vi "manejadorErrores.vi"(8 "error in (no error)":errorcluster, 10 "Enc_values":T1) -> (0 "error out":errorcluster, 2 "Enc_values 2":T1)   [LabVIEW 2026]
uses:
  Control/Ctr_Enc_Values.ctl
  Control/Ctrl_Errores.ctl
  Control/Ctrl_Motores_Valores.ctl
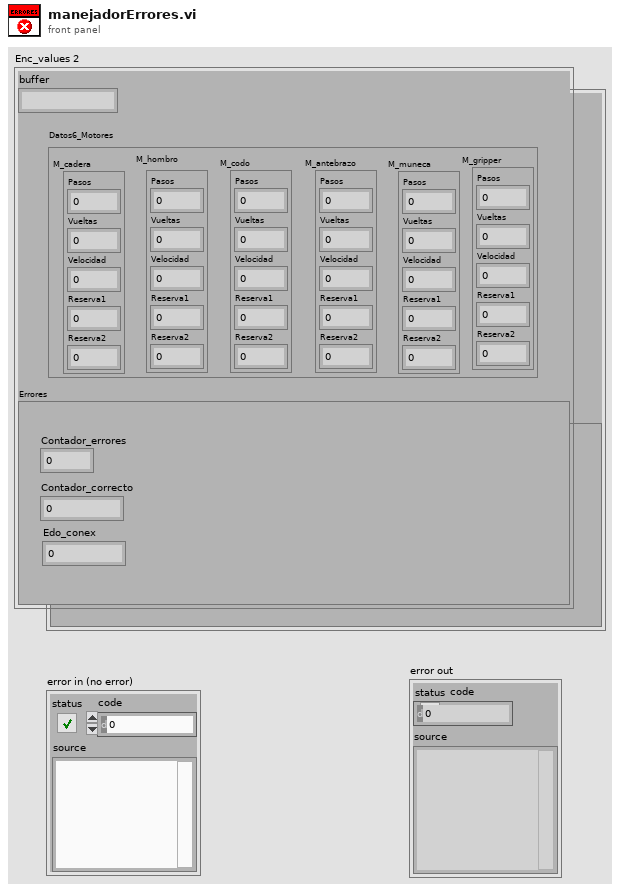
[diagram p1: front panel]
types:
  T1 = typedef "Ctr_Enc_Values.ctl" = cluster{"buffer":string, "Datos6_Motores":cluster{"M_cadera":T2, "M_hombro":T2, "M_codo":T2, "M_antebrazo":T2, "M_muneca":T2, "M_gripper":T2}, "Errores":T3}
  T2 = typedef "Ctrl_Motores_Valores.ctl" = cluster{"Pasos":i32, "Vueltas":i16, "Velocidad":i16, "Reserva1":u8, "Reserva2":u8}
  T3 = typedef "Ctrl_Errores.ctl" = cluster{"Contador_correcto":u32, "Contador_errores":u32, "Edo_conex":u32}
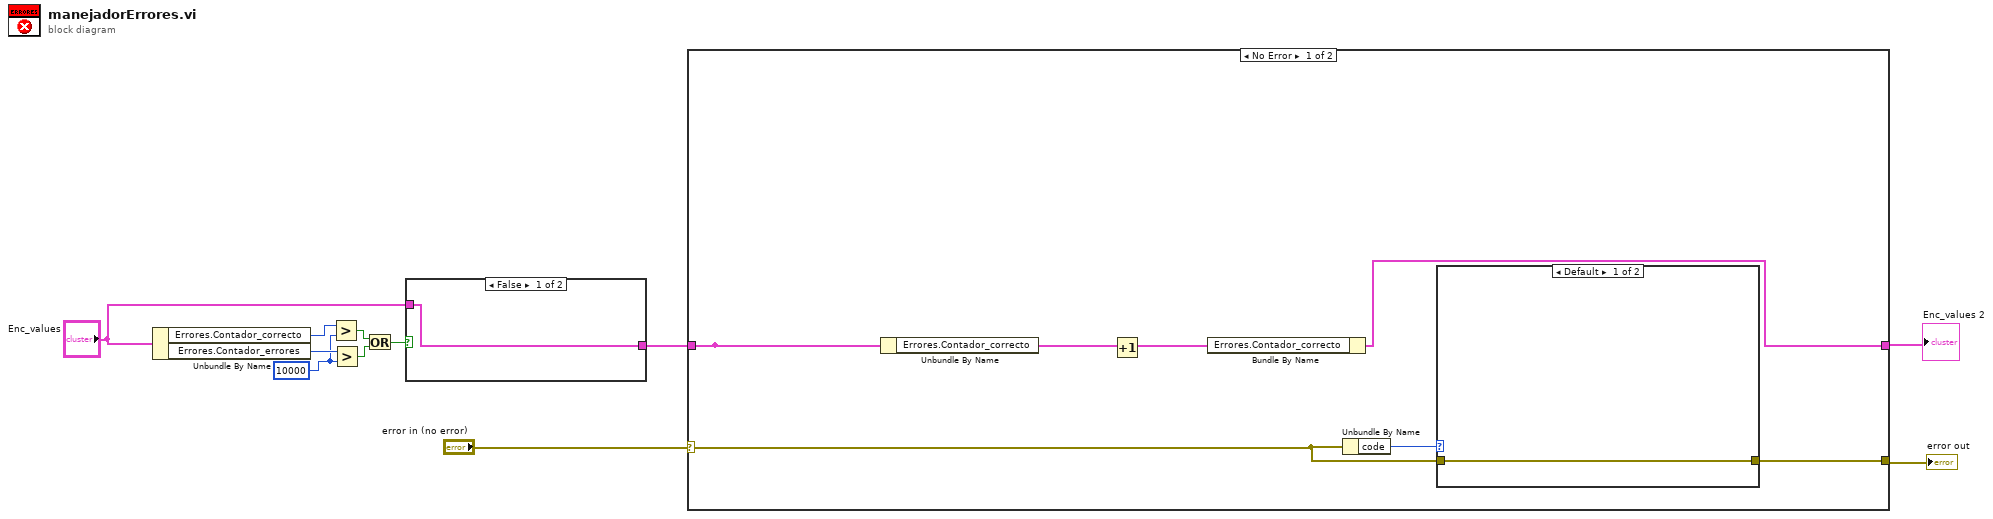
[diagram p0: block diagram]
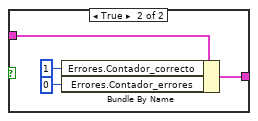
[diagram p2: hidden frame]
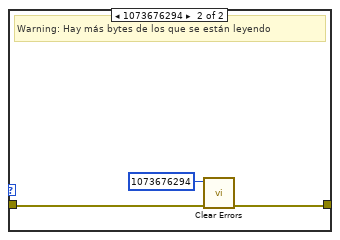
[diagram p3: hidden frame]
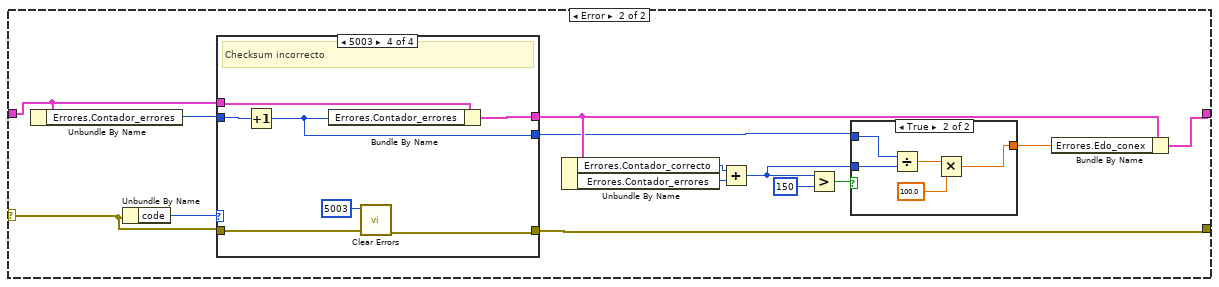
[diagram p4: hidden frame]
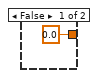
[diagram p5: hidden frame]
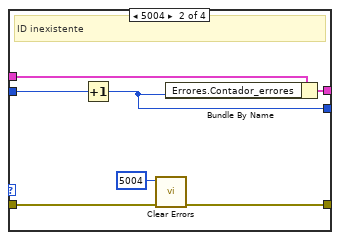
[diagram p7: hidden frame]
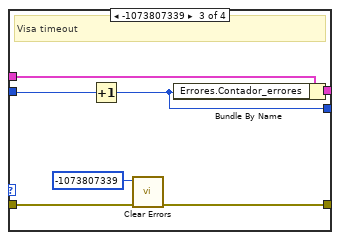
[diagram p8: hidden frame]
diagram:
  w6 = u32 10000 ("y")
  n1 = Unbundle By Name("Enc_values") -> ("Errores.Contador_correcto"=w7:u32, "Errores.Contador_errores"=w8:u32)
  n2 = Greater?(x=w7, y=w6) -> (0:w4:bool)
  n3 = Greater?(x=w8, y=w6) -> (0:w5:bool)
  n4 = Or(x=w4, y=w5) -> (x .or. y?=w3:bool)
  n5 = case shown="False" w3 {
    tunnel: "Enc_values" -> [w12 w16]
    tunnel: [w12 w13] -> w1
    frame False {
    }
    frame True {
      n6 = Bundle By Name(cluster=w16, "Errores.Contador_correcto"=u32 1, "Errores.Contador_errores"=u32 0) -> (w13:T1)
    }
  }
  n7 = case shown="No Error" "error in (no error)" {
    selector: "error in (no error)" -> [w17 w40]
    tunnel: [w19 w39] -> w10
    tunnel: [w20 w37] -> w9
    tunnel: w1 -> [w23 w36]
    frame No Error {
      n8 = Unbundle By Name(w23) -> ("Errores.Contador_correcto"=w21:u32)
      n9 = Increment(x=w21) -> (x+1=w22:u32)
      n10 = Bundle By Name(cluster=w23, "Errores.Contador_correcto"=w22) -> (w20:T1)
      n11 = Unbundle By Name(w17) -> ("code"=w18:i32)
      n12 = case shown="Default" w18 {
        tunnel: w17 -> [w24 w25]
        tunnel: [w24 w26] -> w19
        frame Default {
        }
        frame 1073676294 {
          # "Warning: Hay más bytes de los que se están leyendo"
          n13 = call <vilib>:"Clear Errors.vi"("error in (no error)"=w25, "specific error code to clear (0: all)"=1073676294) -> ("error out"=w26:errorcluster)  [unwired: 4 in, 1 out]
        }
      }
    }
    frame Error {
      n14 = Unbundle By Name(w36) -> ("Errores.Contador_errores"=w35:u32)
      n15 = Unbundle By Name(w40) -> ("code"=w41:i32)
      n16 = case shown="5003" w41 {
        tunnel: w40 -> [w50 w53 w64 w70]
        tunnel: [w50 w54 w63 w69] -> w39
        tunnel: w35 -> [w48 w57 w61 w68]
        tunnel: [w49 w56 w60 w67] -> w38
        tunnel: w36 -> [w49 w52 w59 w66]
        tunnel: [w48 w51 w58 w65] -> w29
        frame Default {
        }
        frame 5004 {
          # "ID inexistente"
          n17 = Increment(x=w57) -> (x+1=w51:u32)
          n18 = call <vilib>:"Clear Errors.vi"("error in (no error)"=w53, "specific error code to clear (0: all)"=5004) -> ("error out"=w54:errorcluster)  [unwired: 4 in, 1 out]
          n19 = Bundle By Name(cluster=w52, "Errores.Contador_errores"=w51) -> (w56:T1)
        }
        frame -1073807339 {
          # "Visa timeout"
          n20 = Increment(x=w61) -> (x+1=w58:u32)
          n21 = call <vilib>:"Clear Errors.vi"("error in (no error)"=w64, "specific error code to clear (0: all)"=-1073807339) -> ("error out"=w63:errorcluster)  [unwired: 4 in, 1 out]
          n22 = Bundle By Name(cluster=w59, "Errores.Contador_errores"=w58) -> (w60:T1)
        }
        frame 5003 {
          # "Checksum incorrecto"
          n23 = Increment(x=w68) -> (x+1=w65:u32)
          n24 = Bundle By Name(cluster=w66, "Errores.Contador_errores"=w65) -> (w67:T1)
          n25 = call <vilib>:"Clear Errors.vi"("error in (no error)"=w70, "specific error code to clear (0: all)"=5003) -> ("error out"=w69:errorcluster)  [unwired: 4 in, 1 out]
        }
      }
      n26 = Unbundle By Name(w38) -> ("Errores.Contador_correcto"=w33:u32, "Errores.Contador_errores"=w34:u32)
      n27 = Add(x=w33, y=w34) -> (x+y=w28:u32)
      n28 = Greater?(x=w28, y=u32 150) -> (0:w31:bool)
      n29 = case shown="True" w31 {
        tunnel: [0.0 w45] -> w30
        tunnel: w29 -> [_ w44]
        tunnel: w28 -> [_ w43]
        frame False {
        }
        frame True {
          n30 = Divide(x=w44, y=w43) -> (x/y=w46:dbl)
          n31 = Multiply(x=w46, y=100.0) -> (x*y=w45:dbl)
        }
      }
      n32 = Bundle By Name(cluster=w38, "Errores.Edo_conex"=w30) -> (w37:T1)
    }
  }
  "error out" <- w10
  "Enc_values 2" <- w9
